vi "ManualTester.vi"() -> ()   [LabVIEW 2015]
uses:
  TronviewGame/VisualizationType.ctl
  TronviewGame/GameRecorder/GameRecorder.lvclass/GameRecorder.ctl
  TronviewGame/GameRecorder/GetInitialBoard.vi
  TronviewGame/GameRecorder/GetPlayer1Name.vi
  TronviewGame/GameRecorder/GetPlayer1Moves.vi
  TronviewGame/GameRecorder/GetPlayer2Name.vi
  TronviewGame/GameRecorder/GetPlayer2Moves.vi
  TronviewGame/Board/Board.lvclass
  TronviewGame/GameRecorder/GameRecorder.lvclass
  TronviewGame/TronviewGame.lvlib
  TronviewGame/Player/Player.lvclass
  ExampleBots/ReplayBot/ReplayBot.lvlib
panel:
  in  "VisualizationType":T1=enum."Simple"
  in  "Game string":string="p1;p2;16,16,0,0,0,0,0,0,0,0,0,0,0,0,0,0,0,0,0,0,0,0,0,0,0,0,0,0,0,0,0,0,0,0,0,0,2,0,0,0,0,0,0,0,0,0,0,0,0,0,0,0,0,0,0,0,0,0,0,0,0,0,0,0,0,0,0,0,0,0,0,0,0,0,0,0,0,0,0,0,0,0,0,0,0,0,0,0,0,0,0,0,0,0,0,0,0,0,0,0,0,0,0,0,0,0,0,0,0,0,0,0,0,0,0,0,0,0,0,0,0,0,0,0,0,0,0,0,0,0,0,0,0,0,0,0,0,0,0,0,0,0,0,0,0,0,0,0,0,0,0,0,0,0,0,0,0,0,0,0,0,0,0,0,0,0,0,0,0,0,0,0,0,0,0,0,0,0,0,0,0,0,0,0,0,0,0,0,0,0,0,0,0,0,0,0,0,0,0,0,0,0,0,0,0,0,0,0,0,0,0,0,0,0,0,0,0,0,0,0,0,0,0,0,0,0,0,0,0,0,0,0,0,0,0,0,0,0,0,0,3,0,0,0,0,0,0,0,0,0,0,0,0,0,0,0,0,0;S,S,S,E,S,W,S,W,N,W,S,S,E,E,S,S,E,N,E,N,E,S,E,S,S,S,E,E,S,W,W,W,W,N,W,W,W,S,W,N,N,E,E,E,E,E,S,S;S,E,N,N,W,W,S,S,W,W,W,W,W,W,W,W,W,W,W,W,W,N,E,E,E,E,E,E,E,E,E,E,E,E,N,W,W,W,N,E,E,E,E,E,E,N,W,W\r\n"
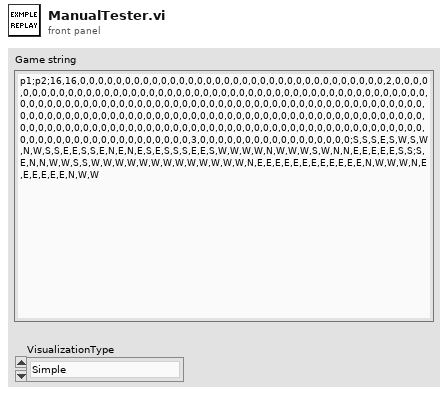
[diagram p1: front panel]
types:
  T1 = typedef "TronviewGame.lvlib/VisualizationType.ctl" = enum16{"None", "Simple", "Fancy"}
  T2 = typedef "TronVIEWBotAPI.lvlib/MovementDirection.ctl" = enum16{"N", "S", "W", "E"}
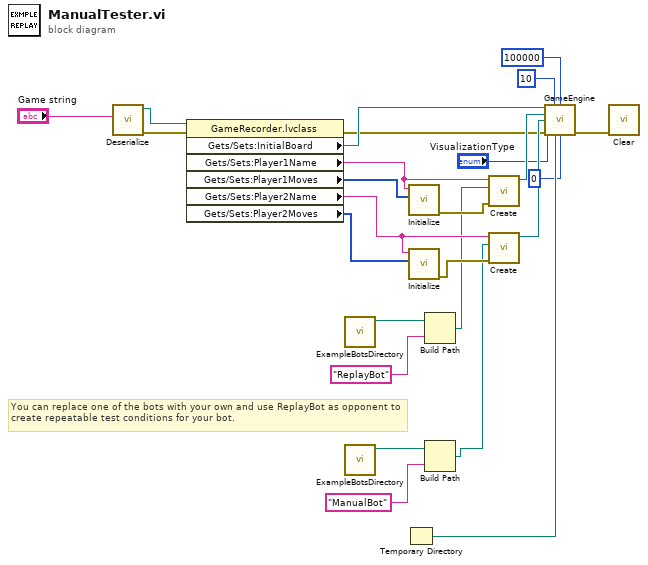
[diagram p0: block diagram]
diagram:
  # "You can replace one of the bots with your own and use ReplayBot as opponent to create repeatable test conditions for your bot."
  n1 = call "Deserialize.vi"("String"="Game string") -> ("error out"=w23:errorcluster, "GameRecorder out"=w24:refnum<class "GameRecorder.lvclass">)  [unwired: 9 in]
  n2 = property class="GameRecorder.lvclass"(reference=w24, error in=w23) -> (error out=w9:errorcluster, "Gets/Sets:InitialBoard"=w22:refnum<class "Board.lvclass">, "Gets/Sets:Player1Name"=w21:string, "Gets/Sets:Player1Moves"=w20:T2[], "Gets/Sets:Player2Name"=w17:string, "Gets/Sets:Player2Moves"=w16:T2[])  [unwired: 1 out]
  n3 = call "ExampleBotsDirectory.vi"() -> ("stripped path"=w12:path)  [unwired: 11 in]
  n4 = call "ExampleBotsDirectory.vi"() -> ("stripped path"=w4:path)  [unwired: 11 in]
  n5 = Temporary Directory() -> (w2:path)
  n6 = call "Initialize.vi"("PlayerMoves"=w20, "PlayerName"=w21) -> ("error out"=w19:errorcluster)  [unwired: 9 in]
  n7 = call "Initialize.vi"("PlayerMoves"=w16, "PlayerName"=w17) -> ("error out"=w18:errorcluster)  [unwired: 9 in]
  n8 = Build Path(base path=w12, name or relative path="ReplayBot") -> (appended path=w10:path)
  n9 = Build Path(base path=w4, name or relative path="ManualBot") -> (appended path=w3:path)
  n10 = call "Create.vi"("error in (no error)"=w19, "PlayerBotFolder"=w10, "PlayerName"=w21) -> ("Player out"=w14:refnum<class "Player.lvclass">)  [unwired: 7 in, 1 out]
  n11 = call "Create.vi"("error in (no error)"=w18, "PlayerBotFolder"=w3, "PlayerName"=w17) -> ("Player out"=w15:refnum<class "Player.lvclass">)  [unwired: 7 in, 1 out]
  n12 = call "GameEngine.vi"("Board"=w22, "IterationDelay (ms)"=u32 10 ("Delay"), "MaxBotProcessingTime (ms)"=100000, "Player1"=w14, "Player2"=w15, "VisualizationType"="VisualizationType", "error in (no error)"=w9, "GameDataFolder"=w2, "MaxBotStorageSize (bytes)"=i64 0) -> ("error out"=w13:errorcluster)  [unwired: 4 in, 2 out]
  n13 = call "Clear.vi"("error in (no error)"=w13) -> ()  [unwired: 10 in, 1 out]
